vi "字符串数组转点坐标.vi"(10 "字符串数组":string[](array[string])) -> (0 "点位坐标XYZR":T1, 2 "点位坐标XYZ":T2)   [LabVIEW 2014]
uses:
  Controls/XYZRPos.ctl
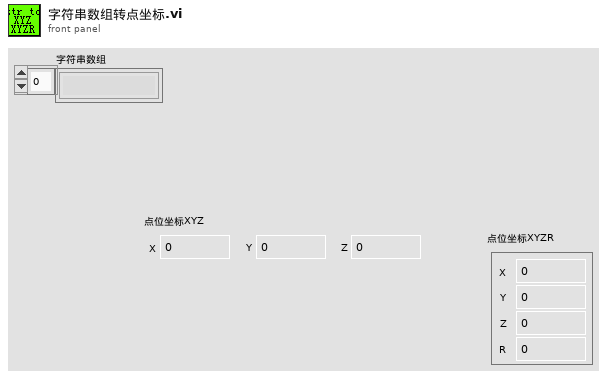
[diagram p1: front panel]
types:
  T1 = typedef "XYZRPos.ctl" = cluster{"X":dbl, "Y":dbl, "Z":dbl, "R":dbl}
  T2 = typedef "锁附点位坐标XYZ.ctl" = cluster{"X":dbl, "Y":dbl, "Z":dbl}
  T3 = cluster{"[0]":dbl, "[1]":dbl, "[2]":dbl, "[3]":dbl}
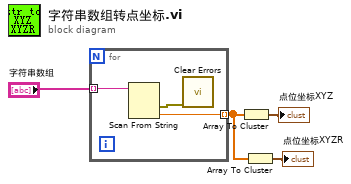
[diagram p0: block diagram]
diagram:
  n1 = for {
    tunnel: "字符串数组" -> [w7] mode=indexing
    tunnel: [w6] -> w1 mode=indexing
    n2 = Scan From String(input string=w7) -> (error out=w5:errorcluster, output 1=w6:dbl)  [unwired: 4 in, 2 out]
    n3 = call <vilib>:"Clear Errors.vi"("error in (no error)"=w5) -> ()  [unwired: 5 in, 2 out]
  }
  n4 = Array To Cluster(array=w1) -> (cluster=→"点位坐标XYZ":cluster{"[0]":dbl, "[1]":dbl, "[2]":dbl})
  n5 = Array To Cluster(array=w1) -> (cluster=→"点位坐标XYZR":T3)
